vi "RSZVB Get Virtual Transform Port Pair Circuit Model.vi"(7 "Port Pair (1)":i32=1, 8 "error in (no error)":errorcluster {"code" format="%.0x"}, 9 "Function Type (Deembedding)":i32(ring) items=["Deembedding", "Embedding"], 10 "Channel (1)":i32=1, 11 "VISA session":refnum<visa-resource-name>) -> (0 "error out":errorcluster {"code" format="%.0x"}, 2 "Circuit Model":i32, 3 "dup VISA session":refnum<visa-resource-name>)   [LabVIEW 2011]
doc: "This VI queries the circuit model for port pair deembedding/embedding.\n\nRemote-control command(s):\nCALCulate<Ch>:TRANsform:VNETworks:PPAir:DEEMbedding<List_idx>:TNDefinition?\nFIMPort | STSL | STSC | SLST | SCST | CSSL | LSSC | CSSC | LSSL | SLCS | SCLS | SCCS | SLLS \nCALCulate<Ch>:TRANsform:VNETworks:PPAir:EMBedding<List_idx>:TNDefinition?\nFIMPort | STSL | STSC | SLST | SCST | CSSL | LSSC | CSSC | LSSL | SLCS | SCLS | SCCS | SLLS"
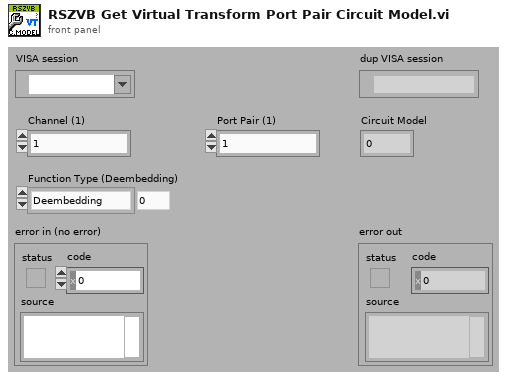
[diagram p1: front panel]
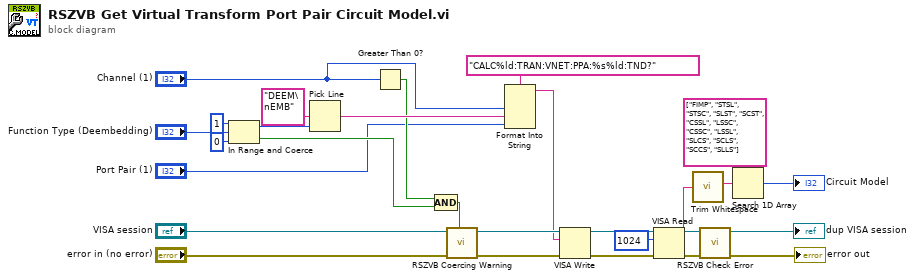
[diagram p0: block diagram]
diagram:
  n1 = In Range and Coerce(upper limit=1, x="Function Type (Deembedding)", lower limit=0) -> (coerced(x)=w23:i32, In Range?=w19:bool)
  n2 = Pick Line(multi-line string="DEEM\nEMB", line index=w23) -> (output string=w22:string)  [unwired: 1 in]
  n3 = Greater Than 0?(x="Channel (1)") -> (x > 0?=w20:bool)
  n4 = Compound Arithmetic op=AND(w20, w19) -> (w18:bool)
  n5 = call "RSZVB Coercing Warning.vi"("In Range?"=w18, "error in (no error)"="error in (no error)", "VISA session"="VISA session") -> ("error out"=w26:errorcluster, "dup VISA session"=w27:refnum<visa-resource-name>)  [unwired: 7 in]
  n6 = Format Into String(format string="CALC%ld:TRAN:VNET:PPA:%s%ld:TND?", "Channel (1)", w22, "Port Pair (1)") -> (resulting string=w21:string)  [unwired: 2 in, 1 out]
  n7 = VISA Write(VISA resource name=w27, write buffer=w21, error in (no error)=w26) -> (VISA resource name out=w7:refnum<visa-resource-name>, error out=w6:errorcluster)  [unwired: 1 out]
  n8 = VISA Read(VISA resource name=w7, byte count=u32 1024 ("byte count (0)"), error in (no error)=w6) -> (VISA resource name out=w12:refnum<visa-resource-name>, read buffer=w8:string, error out=w11:errorcluster)  [unwired: 1 out]
  n9 = call <vilib>:"Trim Whitespace.vi"("string"=w8) -> ("trimmed string"=w10:string)  [unwired: 1 in]
  n10 = call "RSZVB Check Error.vi"("error in (no error)"=w11, "VISA session"=w12) -> ("error out"=→"error out":errorcluster, "dup VISA session"=→"dup VISA session":refnum<visa-resource-name>)  [unwired: 8 in]
  n11 = Search 1D Array(1D array=string[] ["FIMP", "STSL", "STSC", "SLST", "SCST", "CSSL", "LSSC", "CSSC", "LSSL", "SLCS", "SCLS", "SCCS", "SLLS"] ("array 2"), element=w10) -> (index of element=→"Circuit Model":i32)  [unwired: 1 in]
